vi "UT - Label Selectors Write.vi"(11 "Dims":u64[](array[numeric])) -> (1 "Data out":dbl, 2 "Object Types":T1[](array[typedef]) items=["H5G_UNKNOWN"=-1, "H5G_GROUP"=0, "H5G_DATASET"=1, "H5G_TYPE"=2, "H5G_LINK"=3, "H5G_UDLINK"=4], 3 "Object Names":string[](array[string]))   [LabVIEW 2019]
uses:
  <vilib>/UPVI/lvhdf5/group.llb/H5G_obj_t.ctl
  <vilib>/Utility/miscctls.llb/LVRectTypeDef.ctl
  <vilib>/UPVI/lvhdf5/dataset.llb/LVH5D Operation.ctl
  <vilib>/UPVI/lvhdf5/utility.llb/Select HDF5 Dialog.vi
  <vilib>/UPVI/lvhdf5/utility.llb/Select HDF5 Dialog (Object Only).vi
  <vilib>/UPVI/lvhdf5/dataset.llb/Simple H5Dread (Variant).vi
  <vilib>/UPVI/lvhdf5/dataset.llb/Simple H5Dread.xnode
  <vilib>/UPVI/lvhdf5/library.llb/HDF5 Ref.ctl
  HDF5 Tools.lvlib
  <vilib>/UPVI/lvhdf5/file.llb/LVH5F Operation.ctl
  <vilib>/UPVI/lvhdf5/identifier.llb/Not an HDF5 Refnum Constant.vi
  <vilib>/UPVI/lvhdf5/dataset.llb/OpenCreateReplace Dataset.vi
  <vilib>/UPVI/lvhdf5/dataset.llb/H5Dget_space.vi
  <vilib>/UPVI/lvhdf5/dataspace.llb/H5Sget_simple_extent_dims.vi
  <vilib>/UPVI/lvhdf5/dataspace.llb/H5Sselect_hyperslab.vi
  <vilib>/UPVI/lvhdf5/dataset.llb/H5Dread (Variant).vi
  <vilib>/UPVI/lvhdf5/attribute.llb/private/LVH5AreadWDTAttrs.vi
  <vilib>/UPVI/lvhdf5/dataspace.llb/H5Sclose.vi
  <vilib>/Utility/error.llb/Error Cluster From Error Code.vi
  <vilib>/UPVI/lvhdf5/dataset.llb/H5Dclose.vi
  <vilib>/UPVI/lvhdf5/utility.llb/Select HDF5 Dialog (File and Object).vi
panel:
  out "path out":path
  in  "?":T2={"Data"=42.0, "_Attribute"=43.0, "-Skip Me"=44.0}
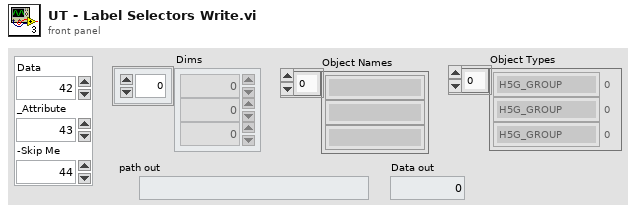
[diagram p1: front panel]
types:
  T1 = typedef "H5G_obj_t.ctl" = i32
  T2 = cluster{"Data":dbl, "_Attribute":dbl, "-Skip Me":dbl}
  T3 = typedef "HDF5 Ref.ctl" = refnum<k1>
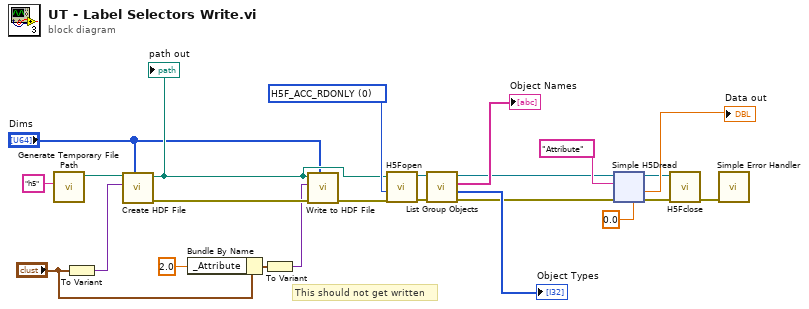
[diagram p0: block diagram]
diagram:
  w19 = u32 0 items=["H5F_ACC_RDONLY", "H5F_ACC_RDWR"] ("flags")
  # "This should not get written"
  n1 = call <vilib>:"Generate Temporary File Path.vi"("Temporary File Extension (tmp)"="h5") -> ("Unique Temporary File Path"=w23:path)  [unwired: 9 in, 1 out]
  n2 = To Variant(anything="?") -> (Variant=w24:variant)
  n3 = call "Create HDF File.vi"("Dims"="Dims", "variant"=w24, "path"=w23) -> ("error out"=w20:errorcluster, "path out"=w4:path)  [unwired: 6 in, 1 out]
  "path out" <- w4
  n4 = Bundle By Name(cluster="?", "_Attribute"=2.0) -> (w3:T2)
  n5 = To Variant(anything=w3) -> (Variant=w1:variant)
  n6 = call "Write to HDF File.vi"("indices"="Dims", "error in (no error)"=w20, "variant"=w1, "path"=w4) -> ("error out"=w5:errorcluster)  [unwired: 7 in]
  n7 = call <vilib>:"H5Fopen.vi"("error in (no error)"=w5, "flags"=w19, "path"=w4) -> ("error out"=w17:errorcluster, "HDF5 Ref out"=w18:T3)  [unwired: 5 in]
  n8 = call <vilib>:"List Group Objects.vi"("error in (no error)"=w17, "HDF5 Loc Ref"=w18) -> ("error out"=w13:errorcluster, "Obect Types"=→"Object Types":T1[], "Object Names"=→"Object Names":string[], "HDF5 Loc Ref out"=w9:T3)  [unwired: 4 in]
  n9 = xnode "Simple H5Dread"("Dataset Path"="Attribute", "error in (no error)"=w13, "HDF5 Path or Ref"=w9, "Data"=0.0) -> ("HDF5 Ref out"=w10:T3, "error out"=w14:errorcluster, "Data out"=→"Data out":dbl)  [unwired: 1 out]
  n10 = call <vilib>:"H5Fclose.vi"("error in (no error)"=w14, "HDF5 Ref"=w10) -> ("error out"=w21:errorcluster)  [unwired: 7 in]
  n11 = call <vilib>:"Simple Error Handler.vi"("error in (no error)"=w21) -> ()  [unwired: 4 in, 5 out]
